vi "nanocal -- nuclear schottky fit V8.vi"() -> ()   [LabVIEW 2021] (continued)
0.000610929623   ,  \"σητS \" -> 0.000000855375   ,  \"σητN\" -> 0.000014389425    |>   , \n\"IDS0370_210908_RAW_cal__sam_\" ->   <|    \"ζ\" -> 0.013427569249   ,  \"τ1\" -> 0.019934074843   ,  \"τS\" -> 0.019524726442   ,  \"τN\" -> 0.000513623253   ,  \"τC\" -> 0.005657316251   ,  \"κ0\" -> 0.000000008143   ,  \"mm1\" -> 0.000058424467   ,  \"mm2\" -> 0.018528796956   ,  \"mm3\" -> 0.027311585694   ,  \"T\" -> 1.130000000000   ,  \"B\" -> 12.000000000000   ,  \"θ\" -> 60.000000000000   ,  \"Reoff\" -> -481927.710843376814   ,  \"Imoff\" -> 0.000000000000   ,  \"στ1\" -> 0.000000000000   ,  \"στS\" -> 0.000000000000   ,  \"στN\" -> 0.000000000000   ,  \"τ11 \" -> 0.000000000000   ,  \"τ12\" -> 0.000000000000   ,  \"τ22\" -> 0.000000000000   ,  \"τN1\" -> 0.000000000000   ,  \"τN2\" -> 0.000000000000   ,  \"σηlogτ1 \" -> 0.000000000000   ,  \"σηlogτS\" -> 0.000000000000   ,  \"σηlogτN\" -> 0.000000000000   ,  \"σlogτ1\" -> 0.000000000000   ,  \"σlogτS\" -> 0.000000000000   ,  \"σlogτN\" -> 0.000000000000   ,  \"σητ1\" -> 0.000000000000   ,  \"σητS \" -> 0.000000000000   ,  \"σητN\" -> 0.000000000000    |>   , \n\"IDS0371_210908_RAW_cal__ref_\" ->   <|    \"ζ\" -> 0.020664849580   ,  \"τ1\" -> 0.018108723176   ,  \"τS\" -> 0.010299896170   ,  \"τN\" -> 0.000079818017   ,  \"τC\" -> 0.006259144045   ,  \"κ0\" -> 0.000000013130   ,  \"mm1\" -> 0.000079811267   ,  \"mm2\" -> 0.016056535433   ,  \"mm3\" -> 0.018825729941   ,  \"T\" -> 1.900000000000   ,  \"B\" -> 12.000000000000   ,  \"θ\" -> 60.000000000000   ,  \"Reoff\" -> 0.000000000000   ,  \"Imoff\" -> 0.000000000000   ,  \"στ1\" -> 0.000000000000   ,  \"στS\" -> 0.000000000000   ,  \"στN\" -> 0.000000000000   ,  \"τ11 \" -> 0.000000000000   ,  \"τ12\" -> 0.000000000000   ,  \"τ22\" -> 0.000000000000   ,  \"τN1\" -> 0.000000000000   ,  \"τN2\" -> 0.000000000000   ,  \"σηlogτ1 \" -> 0.000000000000   ,  \"σηlogτS\" -> 0.000000000000   ,  \"σηlogτN\" -> 0.000000000000   ,  \"σlogτ1\" -> 0.000000000000   ,  \"σlogτS\" -> 0.000000000000   ,  \"σlogτN\" -> 0.000000000000   ,  \"σητ1\" -> 0.000000000000   ,  \"σητS \" -> 0.000000000000   ,  \"σητN\" -> 0.000000000000    |>   , \n\"IDS0371_210908_RAW_cal__sam_\" ->   <|    \"ζ\" -> 0.009645933094   ,  \"τ1\" -> 0.020976887035   ,  \"τS\" -> 0.013140254521   ,  \"τN\" -> 0.000215522697   ,  \"τC\" -> 0.007317042194   ,  \"κ0\" -> 0.000000013897   ,  \"mm1\" -> 0.000045154509   ,  \"mm2\" -> 0.018728618799   ,  \"mm3\" -> 0.023004762073   ,  \"T\" -> 1.900000000000   ,  \"B\" -> 12.000000000000   ,  \"θ\" -> 60.000000000000   ,  \"Reoff\" -> -120481.927710846066   ,  \"Imoff\" -> 0.000000000000   ,  \"στ1\" -> 0.000000000000   ,  \"στS\" -> 0.000000000000   ,  \"στN\" -> 0.000000000000   ,  \"τ11 \" -> 0.000000000000   ,  \"τ12\" -> 0.000000000000   ,  \"τ22\" -> 0.000000000000   ,  \"τN1\" -> 0.000000000000   ,  \"τN2\" -> 0.000000000000   ,  \"σηlogτ1 \" -> 0.000000000000   ,  \"σηlogτS\" -> 0.000000000000   ,  \"σηlogτN\" -> 0.000000000000   ,  \"σlogτ1\" -> 0.000000000000   ,  \"σlogτS\" -> 0.000000000000   ,  \"σlogτN\" -> 0.000000000000   ,  \"σητ1\" -> 0.000000000000   ,  \"σητS \" -> 0.000000000000   ,  \"σητN\" -> 0.000000000000    |>   , \n\"IDS0372_210908_RAW_cal__ref_\" ->   <|    \"ζ\" -> 0.021592146431   ,  \"τ1\" -> 0.018093446545   ,  \"τS\" -> 0.007071841556   ,  \"τN\" -> 0.000029085223   ,  \"τC\" -> 0.005341206531   ,  \"κ0\" -> 0.000000023517   ,  \"mm1\" -> 0.000065243548   ,  \"mm2\" -> 0.012435446609   ,  \"mm3\" -> 0.018188213949   ,  \"T\" -> 3.110000000000   ,  \"B\" -> 12.000000000000   ,  \"θ\" -> 60.000000000000   ,  \"Reoff\" -> 0.000000000000   ,  \"Imoff\" -> 0.000000000000   ,  \"στ1\" -> 0.000000000000   ,  \"στS\" -> 0.000000000000   ,  \"στN\" -> 0.000000000000   ,  \"τ11 \" -> 0.000000000000   ,  \"τ12\" -> 0.000000000000   ,  \"τ22\" -> 0.000000000000   ,  \"τN1\" -> 0.000000000000   ,  \"τN2\" -> 0.000000000000   ,  \"σηlogτ1 \" -> 0.000000000000   ,  \"σηlogτS\" -> 0.000000000000   ,  \"σηlogτN\" -> 0.000000000000   ,  \"σlogτ1\" -> 0.000000000000   ,  \"σlogτS\" -> 0.000000000000   ,  \"σlogτN\" -> 0.000000000000   ,  \"σητ1\" -> 0.000000000000   ,  \"σητS \" -> 0.000000000000   ,  \"σητN\" -> 0.000000000000    |>   , \n\"IDS0372_210908_RAW_cal__sam_\" ->   <|    \"ζ\" -> 0.010006554735   ,  \"τ1\" -> 0.021193289022   ,  \"τS\" -> 0.010059776467   ,  \"τN\" -> 0.000092737128   ,  \"τC\" -> 0.005619947239   ,  \"κ0\" -> 0.000000024358   ,  \"mm1\" -> 0.000035931477   ,  \"mm2\" -> 0.015490366222   ,  \"mm3\" -> 0.021541043840   ,  \"T\" -> 3.110000000000   ,  \"B\" -> 12.000000000000   ,  \"θ\" -> 60.000000000000   ,  \"Reoff\" -> -120481.927710846066   ,  \"Imoff\" -> 0.000000000000   ,  \"στ1\" -> 0.000000000000   ,  \"στS\" -> 0.000000000000   ,  \"στN\" -> 0.000000000000   ,  \"τ11 \" -> 0.000000000000   ,  \"τ12\" -> 0.000000000000   ,  \"τ22\" -> 0.000000000000   ,  \"τN1\" -> 0.000000000000   ,  \"τN2\" -> 0.000000000000   ,  \"σηlogτ1 \" -> 0.000000000000   ,  \"σηlogτS\" -> 0.000000000000   ,  \"σηlogτN\" -> 0.000000000000   ,  \"σlogτ1\" -> 0.000000000000   ,  \"σlogτS\" -> 0.000000000000   ,  \"σlogτN\" -> 0.000000000000   ,  \"σητ1\" -> 0.000000000000   ,  \"σητS \" -> 0.000000000000   ,  \"σητN\" -> 0.000000000000    |>   , \n\"IDS0373_210908_RAW_cal__ref_\" ->   <|    \"ζ\" -> 0.028148688120   ,  \"τ1\" -> 0.012706961955   ,  \"τS\" -> 0.003881518121   ,  \"τN\" -> 0.000007160132   ,  \"τC\" -> 0.004346615253   ,  \"κ0\" -> 0.000000058313   ,  \"mm1\" -> 0.000057355729   ,  \"mm2\" -> 0.008266435527   ,  \"mm3\" -> 0.012727925396   ,  \"T\" -> 5.750000000000   ,  \"B\" -> 12.000000000000   ,  \"θ\" -> 60.000000000000   ,  \"Reoff\" -> 0.000000000000   ,  \"Imoff\" -> 0.000000000000   ,  \"στ1\" -> 0.000000000000   ,  \"στS\" -> 0.000000000000   ,  \"στN\" -> 0.000000000000   ,  \"τ11 \" -> 0.000000000000   ,  \"τ12\" -> 0.000000000000   ,  \"τ22\" -> 0.000000000000   ,  \"τN1\" -> 0.000000000000   ,  \"τN2\" -> 0.000000000000   ,  \"σηlogτ1 \" -> 0.000000000000   ,  \"σηlogτS\" -> 0.000000000000   ,  \"σηlogτN\" -> 0.000000000000   ,  \"σlogτ1\" -> 0.000000000000   ,  \"σlogτS\" -> 0.000000000000   ,  \"σlogτN\" -> 0.000000000000   ,  \"σητ1\" -> 0.000000000000   ,  \"σητS \" -> 0.000000000000   ,  \"σητN\" -> 0.000000000000    |>   , \n\"IDS0373_210908_RAW_cal__sam_\" ->   <|    \"ζ\" -> 0.009383547393   ,  \"τ1\" -> 0.021616814113   ,  \"τS\" -> 0.006389723126   ,  \"τN\" -> 0.000031102862   ,  \"τC\" -> 0.004593168461   ,  \"κ0\" -> 0.000000059183   ,  \"mm1\" -> 0.000024995592   ,  \"mm2\" -> 0.010985466166   ,  \"mm3\" -> 0.021680596929   ,  \"T\" -> 5.750000000000   ,  \"B\" -> 12.000000000000   ,  \"θ\" -> 60.000000000000   ,  \"Reoff\" -> -40000.000000000000   ,  \"Imoff\" -> 0.000000000000   ,  \"στ1\" -> 0.000000000000   ,  \"στS\" -> 0.000000000000   ,  \"στN\" -> 0.000000000000   ,  \"τ11 \" -> 0.000000000000   ,  \"τ12\" -> 0.000000000000   ,  \"τ22\" -> 0.000000000000   ,  \"τN1\" -> 0.000000000000   ,  \"τN2\" -> 0.000000000000   ,  \"σηlogτ1 \" -> 0.000000000000   ,  \"σηlogτS\" -> 0.000000000000   ,  \"σηlogτN\" -> 0.000000000000   ,  \"σlogτ1\" -> 0.000000000000   ,  \"σlogτS\" -> 0.000000000000   ,  \"σlogτN\" -> 0.000000000000   ,  \"σητ1\" -> 0.000000000000   ,  \"σητS \" -> 0.000000000000   ,  \"σητN\" -> 0.000000000000    |>   , \n\"IDS0377_210909_RAW_cal__ref_\" ->   <|    \"ζ\" -> 0.246550605323   ,  \"τ1\" -> 0.063098036224   ,  \"τS\" -> 0.035636106163   ,  \"τN\" -> 0.021974547329   ,  \"τC\" -> 0.000821092988   ,  \"κ0\" -> 0.000000001041   ,  \"mm1\" -> 0.000160015882   ,  \"mm2\" -> 0.025949965723   ,  \"mm3\" -> 0.109623742590   ,  \"T\" -> 0.197000000000   ,  \"B\" -> 8.000000000000   ,  \"θ\" -> 0.000000000000   ,  \"Reoff\" -> -36382320.441988945000   ,  \"Imoff\" -> 0.000000000000   ,  \"στ1\" -> 0.000062922538   ,  \"στS\" -> 0.000014967815   ,  \"στN\" -> 0.000031670740   ,  \"τ11 \" -> 0.000000000000   ,  \"τ12\" -> 0.000000000000   ,  \"τ22\" -> 0.000000000000   ,  \"τN1\" -> 0.000000000000   ,  \"τN2\" -> 0.000000000000   ,  \"σηlogτ1 \" -> 0.000000000000   ,  \"σηlogτS\" -> 0.000000000000   ,  \"σηlogτN\" -> 0.000000000000   ,  \"σlogτ1\" -> 0.000000000000   ,  \"σlogτS\" -> 0.000000000000   ,  \"σlogτN\" -> 0.000000000000   ,  \"σητ1\" -> 0.000000000000   ,  \"σητS \" -> 0.000000000000   ,  \"σητN\" -> 0.000000000000    |>   , \n\"IDS0377_210909_RAW_cal__sam_\" ->   <|    \"ζ\" -> 0.135798490691   ,  \"τ1\" -> 0.079257563336   ,  \"τS\" -> 0.046440970443   ,  \"τN\" -> 0.031537801980   ,  \"τC\" -> 0.001434159670   ,  \"κ0\" -> 0.000000001166   ,  \"mm1\" -> 0.000167444282   ,  \"mm2\" -> 0.031002991367   ,  \"mm3\" -> 0.138089459380   ,  \"T\" -> 0.197000000000   ,  \"B\" -> 8.000000000000   ,  \"θ\" -> 0.000000000000   ,  \"Reoff\" -> -18665662.650602411500   ,  \"Imoff\" -> 0.000000000000   ,  \"στ1\" -> 0.000000000000   ,  \"στS\" -> 0.000000000000   ,  \"στN\" -> 0.000000000000   ,  \"τ11 \" -> 0.000000000000   ,  \"τ12\" -> 0.000000000000   ,  \"τ22\" -> 0.000000000000   ,  \"τN1\" -> 0.000000000000   ,  \"τN2\" -> 0.000000000000   ,  \"σηlogτ1 \" -> 0.000000000000   ,  \"σηlogτS\" -> 0.000000000000   ,  \"σηlogτN\" -> 0.000000000000   ,  \"σlogτ1\" -> 0.000000000000   ,  \"σlogτS\" -> 0.000000000000   ,  \"σlogτN\" -> 0.000000000000   ,  \"σητ1\" -> 0.000000000000   ,  \"σητS \" -> 0.000000000000   ,  \"σητN\" -> 0.000000000000    |>   , \n\"IDS0378_210909_RAW_cal__ref_\" ->   <|    \"ζ\" -> 0.463349829387   ,  \"τ1\" -> 0.074237051581   ,  \"τS\" -> 0.056120726288   ,  \"τN\" -> 0.098410853279   ,  \"τC\" -> 0.000795788528   ,  \"κ0\" -> 0.000000000406   ,  \"mm1\" -> 0.000250303134   ,  \"mm2\" -> 0.022004830152   ,  \"mm3\" -> 0.278911467417   ,  \"T\" -> 0.122000000000   ,  \"B\" -> 8.000000000000   ,  \"θ\" -> 0.000000000000   ,  \"Reoff\" -> -133680722.891566262000   ,  \"Imoff\" -> 0.000000000000   ,  \"στ1\" -> 0.000032928627   ,  \"στS\" -> 0.000022172362   ,  \"στN\" -> 0.000014961504   ,  \"τ11 \" -> 0.000000000000   ,  \"τ12\" -> 0.000000000000   ,  \"τ22\" -> 0.000000000000   ,  \"τN1\" -> 0.000000000000   ,  \"τN2\" -> 0.000000000000   ,  \"σηlogτ1 \" -> 0.000000000000   ,  \"σηlogτS\" -> 0.000000000000   ,  \"σηlogτN\" -> 0.000000000000   ,  \"σlogτ1\" -> 0.000000000000   ,  \"σlogτS\" -> 0.000000000000   ,  \"σlogτN\" -> 0.000000000000   ,  \"σητ1\" -> 0.000000000000   ,  \"σητS \" -> 0.000000000000   ,  \"σητN\" -> 0.000000000000    |>   , \n\"IDS0378_210909_RAW_cal__sam_\" ->   <|    \"ζ\" -> 0.261650469875   ,  \"τ1\" -> 0.181870145043   ,  \"τS\" -> 0.168113301561   ,  \"τN\" -> 0.186965229666   ,  \"τC\" -> 0.001543998203   ,  \"κ0\" -> 0.000000000530   ,  \"mm1\" -> 0.000318362571   ,  \"mm2\" -> 0.069029342513   ,  \"mm3\" -> 0.562051433928   ,  \"T\" -> 0.122000000000   ,  \"B\" -> 8.000000000000   ,  \"θ\" -> 0.000000000000   ,  \"Reoff\" -> -63674698.795180723100   ,  \"Imoff\" -> 0.000000000000   ,  \"στ1\" -> 0.000000000000   ,  \"στS\" -> 0.000000000000   ,  \"στN\" -> 0.000000000000   ,  \"τ11 \" -> 0.000000000000   ,  \"τ12\" -> 0.000000000000   ,  \"τ22\" -> 0.000000000000   ,  \"τN1\" -> 0.000000000000   ,  \"τN2\" -> 0.000000000000   ,  \"σηlogτ1 \" -> 0.000000000000   ,  \"σηlogτS\" -> 0.000000000000   ,  \"σηlogτN\" -> 0.000000000000   ,  \"σlogτ1\" -> 0.000000000000   ,  \"σlogτS\" -> 0.000000000000   ,  \"σlogτN\" -> 0.000000000000   ,  \"σητ1\" -> 0.000000000000   ,  \"σητS \" -> 0.000000000000   ,  \"σητN\" -> 0.000000000000    |>   , \n\"IDS0379_210909_RAW_cal__ref_\" ->   <|    \"ζ\" -> 0.425625100321   ,  \"τ1\" -> 0.068543660714   ,  \"τS\" -> 0.058744737584   ,  \"τN\" -> 0.070392227244   ,  \"τC\" -> 0.000760428296   ,  \"κ0\" -> 0.000000000614   ,  \"mm1\" -> 0.000225582014   ,  \"mm2\" -> 0.025358510497   ,  \"mm3\" -> 0.227820894937   ,  \"T\" -> 0.148000000000   ,  \"B\" -> 8.000000000000   ,  \"θ\" -> 0.000000000000   ,  \"Reoff\" -> -114874585.635359108000   ,  \"Imoff\" -> 0.000000000000   ,  \"στ1\" -> 0.000034854333   ,  \"στS\" -> 0.000021687796   ,  \"στN\" -> 0.000018077177   ,  \"τ11 \" -> 0.000000000000   ,  \"τ12\" -> 0.000000000000   ,  \"τ22\" -> 0.000000000000   ,  \"τN1\" -> 0.000000000000   ,  \"τN2\" -> 0.000000000000   ,  \"σηlogτ1 \" -> 0.000000000000   ,  \"σηlogτS\" -> 0.000000000000   ,  \"σηlogτN\" -> 0.000000000000   ,  \"σlogτ1\" -> 0.000000000000   ,  \"σlogτS\" -> 0.000000000000   ,  \"σlogτN\" -> 0.000000000000   ,  \"σητ1\" -> 0.000000000000   ,  \"σητS \" -> 0.000000000000   ,  \"σητN\" -> 0.000000000000    |>   , \n\"IDS0379_210909_RAW_cal__sam_\" ->   <|    \"ζ\" -> 0.225699737863   ,  \"τ1\" -> 0.105340283181   ,  \"τS\" -> 0.080581728797   ,  \"τN\" -> 0.103261234048   ,  \"τC\" -> 0.001367459466   ,  \"κ0\" -> 0.000000000745   ,  \"mm1\" -> 0.000248975261   ,  \"mm2\" -> 0.035515573270   ,  \"mm3\" -> 0.296279465482   ,  \"T\" -> 0.148000000000   ,  \"B\" -> 8.000000000000   ,  \"θ\" -> 0.000000000000   ,  \"Reoff\" -> -47870481.927710846100   ,  \"Imoff\" -> 0.000000000000   ,  \"στ1\" -> 0.000000000000   ,  \"στS\" -> 0.000000000000   ,  \"στN\" -> 0.000000000000   ,  \"τ11 \" -> 0.000000000000   ,  \"τ12\" -> 0.000000000000   ,  \"τ22\" -> 0.000000000000   ,  \"τN1\" -> 0.000000000000   ,  \"τN2\" -> 0.000000000000   ,  \"σηlogτ1 \" -> 0.000000000000   ,  \"σηlogτS\" -> 0.000000000000   ,  \"σηlogτN\" -> 0.000000000000   ,  \"σlogτ1\" -> 0.000000000000   ,  \"σlogτS\" -> 0.000000000000   ,  \"σlogτN\" -> 0.000000000000   ,  \"σητ1\" -> 0.000000000000   ,  \"σητS \" -> 0.000000000000   ,  \"σητN\" -> 0.000000000000    |>   , \n\"IDS0380_210909_RAW_cal__ref_\" ->   <|    \"ζ\" -> 0.296352280059   ,  \"τ1\" -> 0.061572423860   ,  \"τS\" -> 0.035048599519   ,  \"τN\" -> 0.042254612748   ,  \"τC\" -> 0.000902434218   ,  \"κ0\" -> 0.000000000747   ,  \"mm1\" -> 0.000203161456   ,  \"mm2\" -> 0.019927495587   ,  \"mm3\" -> 0.142556396514   ,  \"T\" -> 0.168000000000   ,  \"B\" -> 8.000000000000   ,  \"θ\" -> 0.000000000000   ,  \"Reoff\" -> -60285714.285714268700   ,  \"Imoff\" -> 0.000000000000   ,  \"στ1\" -> 0.000032565063   ,  \"στS\" -> 0.000015719503   ,  \"στN\" -> 0.000016419375   ,  \"τ11 \" -> 0.000000000000   ,  \"τ12\" -> 0.000000000000   ,  \"τ22\" -> 0.000000000000   ,  \"τN1\" -> 0.000000000000   ,  \"τN2\" -> 0.000000000000   ,  \"σηlogτ1 \" -> 0.000000000000   ,  \"σηlogτS\" -> 0.000000000000   ,  \"σηlogτN\" -> 0.000000000000   ,  \"σlogτ1\" -> 0.000000000000   ,  \"σlogτS\" -> 0.000000000000   ,  \"σlogτN\" -> 0.000000000000   ,  \"σητ1\" -> 0.000000000000   ,  \"σητS \" -> 0.000000000000   ,  \"σητN\" -> 0.000000000000    |>   , \n\"IDS0380_210909_RAW_cal__sam_\" ->   <|    \"ζ\" -> 0.175751625392   ,  \"τ1\" -> 0.093635045165   ,  \"τS\" -> 0.061160146348   ,  \"τN\" -> 0.068664853746   ,  \"τC\" -> 0.001317909381   ,  \"κ0\" -> 0.000000000855   ,  \"mm1\" -> 0.000193962663   ,  \"mm2\" -> 0.031705338902   ,  \"mm3\" -> 0.215695607858   ,  \"T\" -> 0.168000000000   ,  \"B\" -> 8.000000000000   ,  \"θ\" -> 0.000000000000   ,  \"Reoff\" -> -37527108.433734938500   ,  \"Imoff\" -> 0.000000000000   ,  \"στ1\" -> 0.000000000000   ,  \"στS\" -> 0.000000000000   ,  \"στN\" -> 0.000000000000   ,  \"τ11 \" -> 0.000000000000   ,  \"τ12\" -> 0.000000000000   ,  \"τ22\" -> 0.000000000000   ,  \"τN1\" -> 0.000000000000   ,  \"τN2\" -> 0.000000000000   ,  \"σηlogτ1 \" -> 0.000000000000   ,  \"σηlogτS\" -> 0.000000000000   ,  \"σηlogτN\" -> 0.000000000000   ,  \"σlogτ1\" -> 0.000000000000   ,  \"σlogτS\" -> 0.000000000000   ,  \"σlogτN\" -> 0.000000000000   ,  \"σητ1\" -> 0.000000000000   ,  \"σητS \" -> 0.000000000000   ,  \"σητN\" -> 0.000000000000    |>   , \n\"IDS0381_210909_RAW_cal__ref_\" ->   <|    \"ζ\" -> 0.135442001180   ,  \"τ1\" -> 0.054536829593   ,  \"τS\" -> 0.027242617167   ,  \"τN\" -> 0.009575045282   ,  \"τC\" -> 0.001074749120   ,  \"κ0\" -> 0.000000001354   ,  \"mm1\" -> 0.000124377738   ,  \"mm2\" -> 0.023594165009   ,  \"mm3\" -> 0.073697356296   ,  \"T\" -> 0.250000000000   ,  \"B\" -> 8.000000000000   ,  \"θ\" -> 0.000000000000   ,  \"Reoff\" -> -15819277.108433738400   ,  \"Imoff\" -> 0.000000000000   ,  \"στ1\" -> 0.000111598282   ,  \"στS\" -> 0.000013161229   ,  \"στN\" -> 0.000059063513   ,  \"τ11 \" -> 0.000000000000   ,  \"τ12\" -> 0.000000000000   ,  \"τ22\" -> 0.000000000000   ,  \"τN1\" -> 0.000000000000   ,  \"τN2\" -> 0.000000000000   ,  \"σηlogτ1 \" -> 0.000000000000   ,  \"σηlogτS\" -> 0.000000000000   ,  \"σηlogτN\" -> 0.000000000000   ,  \"σlogτ1\" -> 0.000000000000   ,  \"σlogτS\" -> 0.000000000000   ,  \"σlogτN\" -> 0.000000000000   ,  \"σητ1\" -> 0.000000000000   ,  \"σητS \" -> 0.000000000000   ,  \"σητN\" -> 0.000000000000    |>   , \n\"IDS0381_210909_RAW_cal__sam_\" ->   <|    \"ζ\" -> 0.077362618852   ,  \"τ1\" -> 0.058638638627   ,  \"τS\" -> 0.035602410157   ,  \"τN\" -> 0.012932252536   ,  \"τC\" -> 0.001722606032   ,  \"κ0\" -> 0.000000001497   ,  \"mm1\" -> 0.000118727642   ,  \"mm2\" -> 0.027585733079   ,  \"mm3\" -> 0.084946215242   ,  \"T\" -> 0.250000000000   ,  \"B\" -> 8.000000000000   ,  \"θ\" -> 0.000000000000   ,  \"Reoff\" -> -9843373.493975907570   ,  \"Imoff\" -> 0.000000000000   ,  \"στ1\" -> 0.000000000000   ,  \"στS\" -> 0.000000000000   ,  \"στN\" -> 0.000000000000   ,  \"τ11 \" -> 0.000000000000   ,  \"τ12\" -> 0.000000000000   ,  \"τ22\" -> 0.000000000000   ,  \"τN1\" -> 0.000000000000   ,  \"τN2\" -> 0.000000000000   ,  \"σηlogτ1 \" -> 0.000000000000   ,  \"σηlogτS\" -> 0.000000000000   ,  \"σηlogτN\" -> 0.000000000000   ,  \"σlogτ1\" -> 0.000000000000   ,  \"σlogτS\" -> 0.000000000000   ,  \"σlogτN\" -> 0.000000000000   ,  \"σητ1\" -> 0.000000000000   ,  \"σητS \" -> 0.000000000000   ,  \"σητN\" -> 0.000000000000    |>   , \n\"IDS0382_210909_RAW_cal__ref_\" ->   <|    \"ζ\" -> 0.083327700805   ,  \"τ1\" -> 0.049870021008   ,  \"τS\" -> 0.024726462582   ,  \"τN\" -> 0.005137571358   ,  \"τC\" -> 0.001213133652   ,  \"κ0\" -> 0.000000001736   ,  \"mm1\" -> 0.000089554374   ,  \"mm2\" -> 0.023106179536   ,  \"mm3\" -> 0.060239955976   ,  \"T\" -> 0.300000000000   ,  \"B\" -> 8.000000000000   ,  \"θ\" -> 0.000000000000   ,  \"Reoff\" -> -7659638.554216861730   ,  \"Imoff\" -> 0.000000000000   ,  \"στ1\" -> 0.000221537334   ,  \"στS\" -> 0.000014924990   ,  \"στN\" -> 0.000118586370   ,  \"τ11 \" -> 0.000000000000   ,  \"τ12\" -> 0.000000000000   ,  \"τ22\" -> 0.000000000000   ,  \"τN1\" -> 0.000000000000   ,  \"τN2\" -> 0.000000000000   ,  \"σηlogτ1 \" -> 0.000000000000   ,  \"σηlogτS\" -> 0.000000000000   ,  \"σηlogτN\" -> 0.000000000000   ,  \"σlogτ1\" -> 0.000000000000   ,  \"σlogτS\" -> 0.000000000000   ,  \"σlogτN\" -> 0.000000000000   ,  \"σητ1\" -> 0.000000000000   ,  \"σητS \" -> 0.000000000000   ,  \"σητN\" -> 0.000000000000    |>   , \n\"IDS0382_210909_RAW_cal__sam_\" ->   <|    \"ζ\" -> 0.054029770351   ,  \"τ1\" -> 0.051440847518   ,  \"τS\" -> 0.032079834642   ,  \"τN\" -> 0.007150632998   ,  \"τC\" -> 0.002202148776   ,  \"κ0\" -> 0.000000001884   ,  \"mm1\" -> 0.000106291219   ,  \"mm2\" -> 0.027352636275   ,  \"mm3\" -> 0.067534149597   ,  \"T\" -> 0.300000000000   ,  \"B\" -> 8.000000000000   ,  \"θ\" -> 0.000000000000   ,  \"Reoff\" -> 0.000000000000   ,  \"Imoff\" -> 0.000000000000   ,  \"στ1\" -> 0.000000000000   ,  \"στS\" -> 0.000000000000   ,  \"στN\" -> 0.000000000000   ,  \"τ11 \" -> 0.000000000000   ,  \"τ12\" -> 0.000000000000   ,  \"τ22\" -> 0.000000000000   ,  \"τN1\" -> 0.000000000000   ,  \"τN2\" -> 0.000000000000   ,  \"σηlogτ1 \" -> 0.000000000000   ,  \"σηlogτS\" -> 0.000000000000   ,  \"σηlogτN\" -> 0.000000000000   ,  \"σlogτ1\" -> 0.000000000000   ,  \"σlogτS\" -> 0.000000000000   ,  \"σlogτN\" -> 0.000000000000   ,  \"σητ1\" -> 0.000000000000   ,  \"σητS \" -> 0.000000000000   ,  \"σητN\" -> 0.000000000000    |>   , \n\"IDS0383_210910_RAW_cal__ref_\" ->   <|    \"ζ\" -> 0.062724752087   ,  \"τ1\" -> 0.048607141774   ,  \"τS\" -> 0.023827543799   ,  \"τN\" -> 0.003390848411   ,  \"τC\" -> 0.001761568500   ,  \"κ0\" -> 0.000000002107   ,  \"mm1\" -> 0.000097559485   ,  \"mm2\" -> 0.023589285914   ,  \"mm3\" -> 0.055607523989   ,  \"T\" -> 0.360000000000   ,  \"B\" -> 8.000000000000   ,  \"θ\" -> 0.000000000000   ,  \"Reoff\" -> -3448979.591836734680   ,  \"Imoff\" -> 0.000000000000   ,  \"στ1\" -> 0.000376669141   ,  \"στS\" -> 0.000017301947   ,  \"στN\" -> 0.000201176295   ,  \"τ11 \" -> 0.000000000000   ,  \"τ12\" -> 0.000000000000   ,  \"τ22\" -> 0.000000000000   ,  \"τN1\" -> 0.000000000000   ,  \"τN2\" -> 0.000000000000   ,  \"σηlogτ1 \" -> 0.000000000000   ,  \"σηlogτS\" -> 0.000000000000   ,  \"σηlogτN\" -> 0.000000000000   ,  \"σlogτ1\" -> 0.000000000000   ,  \"σlogτS\" -> 0.000000000000   ,  \"σlogτN\" -> 0.000000000000   ,  \"σητ1\" -> 0.000000000000   ,  \"σητS \" -> 0.000000000000   ,  \"σητN\" -> 0.000000000000    |>   , \n\"IDS0383_210910_RAW_cal__sam_\" ->   <|    \"ζ\" -> 0.038341835326   ,  \"τ1\" -> 0.050866858713   ,  \"τS\" -> 0.030652081909   ,  \"τN\" -> 0.004623805952   ,  \"τC\" -> 0.002823684758   ,  \"κ0\" -> 0.000000002289   ,  \"mm1\" -> 0.000096034779   ,  \"mm2\" -> 0.028459102290   ,  \"mm3\" -> 0.061763836547   ,  \"T\" -> 0.360000000000   ,  \"B\" -> 8.000000000000   ,  \"θ\" -> 0.000000000000   ,  \"Reoff\" -> 0.000000000000   ,  \"Imoff\" -> 0.000000000000   ,  \"στ1\" -> 0.000000000000   ,  \"στS\" -> 0.000000000000   ,  \"στN\" -> 0.000000000000   ,  \"τ11 \" -> 0.000000000000   ,  \"τ12\" -> 0.000000000000   ,  \"τ22\" -> 0.000000000000   ,  \"τN1\" -> 0.000000000000   ,  \"τN2\" -> 0.000000000000   ,  \"σηlogτ1 \" -> 0.000000000000   ,  \"σηlogτS\" -> 0.000000000000   ,  \"σηlogτN\" -> 0.000000000000   ,  \"σlogτ1\" -> 0.000000000000   ,  \"σlogτS\" -> 0.000000000000   ,  \"σlogτN\" -> 0.000000000000   ,  \"σητ1\" -> 0.000000000000   ,  \"σητS \" -> 0.000000000000   ,  \"σητN\" -> 0.000000000000    |>   , \n\"IDS0384_210910_RAW_cal__ref_\" ->   <|    \"ζ\" -> 0.048414028377   ,  \"τ1\" -> 0.045010611313   ,  \"τS\" -> 0.024057574241   ,  \"τN\" -> 0.002275401127   ,  \"τC\" -> 0.001753445489   ,  \"κ0\" -> 0.000000002628   ,  \"mm1\" -> 0.000075920940   ,  \"mm2\" -> 0.024140914114   ,  \"mm3\" -> 0.050155082533   ,  \"T\" -> 0.430000000000   ,  \"B\" -> 8.000000000000   ,  \"θ\" -> 0.000000000000   ,  \"Reoff\" -> -3244897.959183673380   ,  \"Imoff\" -> 0.000000000000   ,  \"στ1\" -> 0.000665063032   ,  \"στS\" -> 0.000021368158   ,  \"στN\" -> 0.000342578343   ,  \"τ11 \" -> 0.000000000000   ,  \"τ12\" -> 0.000000000000   ,  \"τ22\" -> 0.000000000000   ,  \"τN1\" -> 0.000000000000   ,  \"τN2\" -> 0.000000000000   ,  \"σηlogτ1 \" -> 0.000000000000   ,  \"σηlogτS\" -> 0.000000000000   ,  \"σηlogτN\" -> 0.000000000000   ,  \"σlogτ1\" -> 0.000000000000   ,  \"σlogτS\" -> 0.000000000000   ,  \"σlogτN\" -> 0.000000000000   ,  \"σητ1\" -> 0.000000000000   ,  \"σητS \" -> 0.000000000000   ,  \"σητN\" -> 0.000000000000    |>   , \n\"IDS0384_210910_RAW_cal__sam_\" ->   <|    \"ζ\" -> 0.029950572027   ,  \"τ1\" -> 0.044923259835   ,  \"τS\" -> 0.030416367718   ,  \"τN\" -> 0.002541256331   ,  \"τC\" -> 0.003331031560   ,  \"κ0\" -> 0.000000002858   ,  \"mm1\" -> 0.000087776347   ,  \"mm2\" -> 0.029544080465   ,  \"mm3\" -> 0.052567158325   ,  \"T\" -> 0.430000000000   ,  \"B\" -> 8.000000000000   ,  \"θ\" -> 0.000000000000   ,  \"Reoff\" -> 0.000000000000   ,  \"Imoff\" -> 0.000000000000   ,  \"στ1\" -> 0.000000000000   ,  \"στS\" -> 0.000000000000   ,  \"στN\" -> 0.000000000000   ,  \"τ11 \" -> 0.000000000000   ,  \"τ12\" -> 0.000000000000   ,  \"τ22\" -> 0.000000000000   ,  \"τN1\" -> 0.000000000000   ,  \"τN2\" -> 0.000000000000   ,  \"σηlogτ1 \" -> 0.000000000000   ,  \"σηlogτS\" -> 0.000000000000   ,  \"σηlogτN\" -> 0.000000000000   ,  \"σlogτ1\" -> 0.000000000000   ,  \"σlogτS\" -> 0.000000000000   ,  \"σlogτN\" -> 0.000000000000   ,  \"σητ1\" -> 0.000000000000   ,  \"σητS \" -> 0.000000000000   ,  \"σητN\" -> 0.000000000000    |>   , \n\"IDS0385_210910_RAW_cal__ref_\" ->   <|    \"ζ\" -> 0.037803233744   ,  \"τ1\" -> 0.038048590559   ,  \"τS\" -> 0.025073667725   ,  \"τN\" -> 0.001214857209   ,  \"τC\" -> 0.002021423784   ,  \"κ0\" -> 0.000000003274   ,  \"mm1\" -> 0.000068491984   ,  \"mm2\" -> 0.025433188254   ,  \"mm3\" -> 0.041850650292   ,  \"T\" -> 0.530000000000   ,  \"B\" -> 8.000000000000   ,  \"θ\" -> 0.000000000000   ,  \"Reoff\" -> -1979591.836734693500   ,  \"Imoff\" -> 0.000000000000   ,  \"στ1\" -> 0.001496353936   ,  \"στS\" -> 0.000028774209   ,  \"στN\" -> 0.000698641170   ,  \"τ11 \" -> 0.000000000000   ,  \"τ12\" -> 0.000000000000   ,  \"τ22\" -> 0.000000000000   ,  \"τN1\" -> 0.000000000000   ,  \"τN2\" -> 0.000000000000   ,  \"σηlogτ1 \" -> 0.000000000000   ,  \"σηlogτS\" -> 0.000000000000   ,  \"σηlogτN\" -> 0.000000000000   ,  \"σlogτ1\" -> 0.000000000000   ,  \"σlogτS\" -> 0.000000000000   ,  \"σlogτN\" -> 0.000000000000   ,  \"σητ1\" -> 0.000000000000   ,  \"σητS \" -> 0.000000000000   ,  \"σητN\" -> 0.000000000000    |>   , \n\"IDS0385_210910_RAW_cal__sam_\" ->   <|    \"ζ\" -> 0.024600756648   ,  \"τ1\" -> 0.043958236582   ,  \"τS\" -> 0.031312750224   ,  \"τN\" -> 0.001348105931   ,  \"τC\" -> 0.003635120795   ,  \"κ0\" -> 0.000000003548   ,  \"mm1\" -> 0.000078569164   ,  \"mm2\" -> 0.031960914170   ,  \"mm3\" -> 0.049018211972   ,  \"T\" -> 0.530000000000   ,  \"B\" -> 8.000000000000   ,  \"θ\" -> 0.000000000000   ,  \"Reoff\" -> 0.000000000000   ,  \"Imoff\" -> 0.000000000000   ,  \"στ1\" -> 0.000000000000   ,  \"στS\" -> 0.000000000000   ,  \"στN\" -> 0.000000000000   ,  \"τ11 \" -> 0.000000000000   ,  \"τ12\" -> 0.000000000000   ,  \"τ22\" -> 0.000000000000   ,  \"τN1\" -> 0.000000000000   ,  \"τN2\" -> 0.000000000000   ,  \"σηlogτ1 \" -> 0.000000000000   ,  \"σηlogτS\" -> 0.000000000000   ,  \"σηlogτN\" -> 0.000000000000   ,  \"σlogτ1\" -> 0.000000000000   ,  \"σlogτS\" -> 0.000000000000   ,  \"σlogτN\" -> 0.000000000000   ,  \"σητ1\" -> 0.000000000000   ,  \"σητS \" -> 0.000000000000   ,  \"σητN\" -> 0.000000000000    |>   , \n\"IDS0386_210910_RAW_cal__ref_\" ->   <|    \"ζ\" -> 0.027746649612   ,  \"τ1\" -> 0.033747008640   ,  \"τS\" -> 0.026895844648   ,  \"τN\" -> 0.000802809162   ,  \"τC\" -> 0.002381968002   ,  \"κ0\" -> 0.000000003893   ,  \"mm1\" -> 0.000059322452   ,  \"mm2\" -> 0.026788808143   ,  \"mm3\" -> 0.037748044699   ,  \"T\" -> 0.630000000000   ,  \"B\" -> 8.000000000000   ,  \"θ\" -> 0.000000000000   ,  \"Reoff\" -> -918367.346938774919   ,  \"Imoff\" -> 0.000000000000   ,  \"στ1\" -> 0.002776813512   ,  \"στS\" -> 0.000037245612   ,  \"στN\" -> 0.001225903353   ,  \"τ11 \" -> 0.000000000000   ,  \"τ12\" -> 0.000000000000   ,  \"τ22\" -> 0.000000000000   ,  \"τN1\" -> 0.000000000000   ,  \"τN2\" -> 0.000000000000   ,  \"σηlogτ1 \" -> 0.000000000000   ,  \"σηlogτS\" -> 0.000000000000   ,  \"σηlogτN\" -> 0.000000000000   ,  \"σlogτ1\" -> 0.000000000000   ,  \"σlogτS\" -> 0.000000000000   ,  \"σlogτN\" -> 0.000000000000   ,  \"σητ1\" -> 0.000000000000   ,  \"σητS \" -> 0.000000000000   ,  \"σητN\" -> 0.000000000000    |>   , \n\"IDS0386_210910_RAW_cal__sam_\" ->   <|    \"ζ\" -> 0.019494767421   ,  \"τ1\" -> 0.040349410363   ,  \"τS\" -> 0.033202805363   ,  \"τN\" -> 0.000770756985   ,  \"τC\" -> 0.004303152006   ,  \"κ0\" -> 0.000000004241   ,  \"mm1\" -> 0.000073144130   ,  \"mm2\" -> 0.033928832906   ,  \"mm3\" -> 0.045286454378   ,  \"T\" -> 0.630000000000   ,  \"B\" -> 8.000000000000   ,  \"θ\" -> 0.000000000000   ,  \"Reoff\" -> 0.000000000000   ,  \"Imoff\" -> 0.000000000000   ,  \"στ1\" -> 0.000000000000   ,  \"στS\" -> 0.000000000000   ,  \"στN\" -> 0.000000000000   ,  \"τ11 \" -> 0.000000000000   ,  \"τ12\" -> 0.000000000000   ,  \"τ22\" -> 0.000000000000   ,  \"τN1\" -> 0.000000000000   ,  \"τN2\" -> 0.000000000000   ,  \"σηlogτ1 \" -> 0.000000000000   ,  \"σηlogτS\" -> 0.000000000000   ,  \"σηlogτN\" -> 0.000000000000   ,  \"σlogτ1\" -> 0.000000000000   ,  \"σlogτS\" -> 0.000000000000   ,  \"σlogτN\" -> 0.000000000000   ,  \"σητ1\" -> 0.000000000000   ,  \"σητS \" -> 0.000000000000   ,  \"σητN\" -> 0.000000000000    |>   , \n\"IDS0387_210910_RAW_cal__ref_\" ->   <|    \"ζ\" -> 0.019313601846   ,  \"τ1\" -> 0.030127940029   ,  \"τS\" -> 0.030834079671   ,  \"τN\" -> 0.000314036282   ,  \"τC\" -> 0.003752610189   ,  \"κ0\" -> 0.000000005418   ,  \"mm1\" -> 0.000063634095   ,  \"mm2\" -> 0.028697652257   ,  \"mm3\" -> 0.036868962129   ,  \"T\" -> 0.830000000000   ,  \"B\" -> 8.000000000000   ,  \"θ\" -> 0.000000000000   ,  \"Reoff\" -> -265306.122448978945   ,  \"Imoff\" -> 0.000000000000   ,  \"στ1\" -> 0.011424377975   ,  \"στS\" -> 0.000061541841   ,  \"στN\" -> 0.005052534408   ,  \"τ11 \" -> 0.000000000000   ,  \"τ12\" -> 0.000000000000   ,  \"τ22\" -> 0.000000000000   ,  \"τN1\" -> 0.000000000000   ,  \"τN2\" -> 0.000000000000   ,  \"σηlogτ1 \" -> 0.000000000000   ,  \"σηlogτS\" -> 0.000000000000   ,  \"σηlogτN\" -> 0.000000000000   ,  \"σlogτ1\" -> 0.000000000000   ,  \"σlogτS\" -> 0.000000000000   ,  \"σlogτN\" -> 0.000000000000   ,  \"σητ1\" -> 0.000000000000   ,  \"σητS \" -> 0.000000000000   ,  \"σητN\" -> 0.000000000000    |>   , \n\"IDS0387_210910_RAW_cal__sam_\" ->   <|    \"ζ\" -> 0.013958531253   ,  \"τ1\" -> 0.040449551738   ,  \"τS\" -> 0.038075316972   ,  \"τN\" -> 0.000218997482   ,  \"τC\" -> 0.005348147372   ,  \"κ0\" -> 0.000000005866   ,  \"mm1\" -> 0.000064761782   ,  \"mm2\" -> 0.038768935960   ,  \"mm3\" -> 0.045792848207   ,  \"T\" -> 0.830000000000   ,  \"B\" -> 8.000000000000   ,  \"θ\" -> 0.000000000000   ,  \"Reoff\" -> 0.000000000000   ,  \"Imoff\" -> 0.000000000000   ,  \"στ1\" -> 0.000000000000   ,  \"στS\" -> 0.000000000000   ,  \"στN\" -> 0.000000000000   ,  \"τ11 \" -> 0.000000000000   ,  \"τ12\" -> 0.000000000000   ,  \"τ22\" -> 0.000000000000   ,  \"τN1\" -> 0.000000000000   ,  \"τN2\" -> 0.000000000000   ,  \"σηlogτ1 \" -> 0.000000000000   ,  \"σηlogτS\" -> 0.000000000000   ,  \"σηlogτN\" -> 0.000000000000   ,  \"σlogτ1\" -> 0.000000000000   ,  \"σlogτS\" -> 0.000000000000   ,  \"σlogτN\" -> 0.000000000000   ,  \"σητ1\" -> 0.000000000000   ,  \"σητS \" -> 0.000000000000   ,  \"σητN\" -> 0.000000000000    |>   , \n\"IDS0388_210910_RAW_cal__ref_\" ->   <|    \"ζ\" -> 0.016319215592   ,  \"τ1\" -> 0.028476907475   ,  \"τS\" -> 0.040634863110   ,  \"τN\" -> 0.000119778793   ,  \"τC\" -> 0.003363489331   ,  \"κ0\" -> 0.000000007540   ,  \"mm1\" -> 0.000049996694   ,  \"mm2\" -> 0.028266417043   ,  \"mm3\" -> 0.044943708759   ,  \"T\" -> 1.130000000000   ,  \"B\" -> 8.000000000000   ,  \"θ\" -> 0.000000000000   ,  \"Reoff\" -> -428571.428571428172   ,  \"Imoff\" -> 0.000000000000   ,  \"στ1\" -> 0.056097814520   ,  \"στS\" -> 0.000101338732   ,  \"στN\" -> 0.027741009439   ,  \"τ11 \" -> 0.000000000000   ,  \"τ12\" -> 0.000000000000   ,  \"τ22\" -> 0.000000000000   ,  \"τN1\" -> 0.000000000000   ,  \"τN2\" -> 0.000000000000   ,  \"σηlogτ1 \" -> 0.000000000000   ,  \"σηlogτS\" -> 0.000000000000   ,  \"σηlogτN\" -> 0.000000000000   ,  \"σlogτ1\" -> 0.000000000000   ,  \"σlogτS\" -> 0.000000000000   ,  \"σlogτN\" -> 0.000000000000   ,  \"σητ1\" -> 0.000000000000   ,  \"σητS \" -> 0.000000000000   ,  \"σητN\" -> 0.000000000000    |>   , \n\"IDS0388_210910_RAW_cal__sam_\" ->   <|    \"ζ\" -> 0.011551866824   ,  \"τ1\" -> 0.040411227639   ,  \"τS\" -> 0.048181354691   ,  \"τN\" -> 0.000103559724   ,  \"τC\" -> 0.006232382617   ,  \"κ0\" -> 0.000000008161   ,  \"mm1\" -> 0.000063176601   ,  \"mm2\" -> 0.040126882627   ,  \"mm3\" -> 0.055296246344   ,  \"T\" -> 1.130000000000   ,  \"B\" -> 8.000000000000   ,  \"θ\" -> 0.000000000000   ,  \"Reoff\" -> 0.000000000000   ,  \"Imoff\" -> 0.000000000000   ,  \"στ1\" -> 0.000000000000   ,  \"στS\" -> 0.000000000000   ,  \"στN\" -> 0.000000000000   ,  \"τ11 \" -> 0.000000000000   ,  \"τ12\" -> 0.000000000000   ,  \"τ22\" -> 0.000000000000   ,  \"τN1\" -> 0.000000000000   ,  \"τN2\" -> 0.000000000000   ,  \"σηlogτ1 \" -> 0.000000000000   ,  \"σηlogτS\" -> 0.000000000000   ,  \"σηlogτN\" -> 0.000000000000   ,  \"σlogτ1\" -> 0.000000000000   ,  \"σlogτS\" -> 0.000000000000   ,  \"σlogτN\" -> 0.000000000000   ,  \"σητ1\" -> 0.000000000000   ,  \"σητS \" -> 0.000000000000   ,  \"σητN\" -> 0.000000000000    |>   , \n\"IDS0389_210910_RAW_cal__ref_\" ->   <|    \"ζ\" -> 0.019598304636   ,  \"τ1\" -> 0.026919422871   ,  \"τS\" -> 0.016301457757   ,  \"τN\" -> 0.000045685674   ,  \"τC\" -> 0.003967911941   ,  \"κ0\" -> 0.000000010417   ,  \"mm1\" -> 0.000061755971   ,  \"mm2\" -> 0.020381971483   ,  \"mm3\" -> 0.027111127086   ,  \"T\" -> 1.520000000000   ,  \"B\" -> 8.000000000000   ,  \"θ\" -> 0.000000000000   ,  \"Reoff\" -> -551020.408163265324   ,  \"Imoff\" -> 0.000000000000   ,  \"στ1\" -> 0.092677427953   ,  \"στS\" -> 0.000105745650   ,  \"στN\" -> 0.043266676347   ,  \"τ11 \" -> 0.000000000000   ,  \"τ12\" -> 0.000000000000   ,  \"τ22\" -> 0.000000000000   ,  \"τN1\" -> 0.000000000000   ,  \"τN2\" -> 0.000000000000   ,  \"σηlogτ1 \" -> 0.000000000000   ,  \"σηlogτS\" -> 0.000000000000   ,  \"σηlogτN\" -> 0.000000000000   ,  \"σlogτ1\" -> 0.000000000000   ,  \"σlogτS\" -> 0.000000000000   ,  \"σlogτN\" -> 0.000000000000   ,  \"σητ1\" -> 0.000000000000   ,  \"σητS \" -> 0.000000000000   ,  \"σητN\" -> 0.000000000000    |>   , \n\"IDS0389_210910_RAW_cal__sam_\" ->   <|    \"ζ\" -> 0.011148198813   ,  \"τ1\" -> 0.038849151842   ,  \"τS\" -> 0.019213865355   ,  \"τN\" -> 0.000045035153   ,  \"τC\" -> 0.005536708133   ,  \"κ0\" -> 0.000000011229   ,  \"mm1\" -> 0.000047596165   ,  \"mm2\" -> 0.024836509281   ,  \"mm3\" -> 0.038975357089   ,  \"T\" -> 1.520000000000   ,  \"B\" -> 8.000000000000   ,  \"θ\" -> 0.000000000000   ,  \"Reoff\" -> 0.000000000000   ,  \"Imoff\" -> 0.000000000000   ,  \"στ1\" -> 0.000000000000   ,  \"στS\" -> 0.000000000000   ,  \"στN\" -> 0.000000000000   ,  \"τ11 \" -> 0.000000000000   ,  \"τ12\" -> 0.000000000000   ,  \"τ22\" -> 0.000000000000   ,  \"τN1\" -> 0.000000000000   ,  \"τN2\" -> 0.000000000000   ,  \"σηlogτ1 \" -> 0.000000000000   ,  \"σηlogτS\" -> 0.000000000000   ,  \"σηlogτN\" -> 0.000000000000   ,  \"σlogτ1\" -> 0.000000000000   ,  \"σlogτS\" -> 0.000000000000   ,  \"σlogτN\" -> 0.000000000000   ,  \"σητ1\" -> 0.000000000000   ,  \"σητS \" -> 0.000000000000   ,  \"σητN\" -> 0.000000000000    |>   , \n\"IDS0390_210910_RAW_cal__ref_\" ->   <|    \"ζ\" -> 0.016930911493   ,  \"τ1\" -> 0.024035041541   ,  \"τS\" -> 0.011182752166   ,  \"τN\" -> 0.000024854278   ,  \"τC\" -> 0.003445627696   ,  \"κ0\" -> 0.000000013051   ,  \"mm1\" -> 0.000044158259   ,  \"mm2\" -> 0.014733556006   ,  \"mm3\" -> 0.024100316408   ,  \"T\" -> 1.900000000000   ,  \"B\" -> 8.000000000000   ,  \"θ\" -> 0.000000000000   ,  \"Reoff\" -> -346938.775510204024   ,  \"Imoff\" -> 0.000000000000   ,  \"στ1\" -> 0.156695414704   ,  \"στS\" -> 0.000120966838   ,  \"στN\" -> 0.078791038522   ,  \"τ11 \" -> 0.000000000000   ,  \"τ12\" -> 0.000000000000   ,  \"τ22\" -> 0.000000000000   ,  \"τN1\" -> 0.000000000000   ,  \"τN2\" -> 0.000000000000   ,  \"σηlogτ1 \" -> 0.000000000000   ,  \"σηlogτS\" -> 0.000000000000   ,  \"σηlogτN\" -> 0.000000000000   ,  \"σlogτ1\" -> 0.000000000000   ,  \"σlogτS\" -> 0.000000000000   ,  \"σlogτN\" -> 0.000000000000   ,  \"σητ1\" -> 0.000000000000   ,  \"σητS \" -> 0.000000000000   ,  \"σητN\" -> 0.000000000000    |>   , \n\"IDS0390_210910_RAW_cal__sam_\" ->   <|    \"ζ\" -> 0.010826949430   ,  \"τ1\" -> 0.038768037521   ,  \"τS\" -> 0.012925317198   ,  \"τN\" -> 0.000029157336   ,  \"τC\" -> 0.005196063884   ,  \"κ0\" -> 0.000000013864   ,  \"mm1\" -> 0.000039906108   ,  \"mm2\" -> 0.018195372076   ,  \"mm3\" -> 0.038823555195   ,  \"T\" -> 1.900000000000   ,  \"B\" -> 8.000000000000   ,  \"θ\" -> 0.000000000000   ,  \"Reoff\" -> 0.000000000000   ,  \"Imoff\" -> 0.000000000000   ,  \"στ1\" -> 0.000000000000   ,  \"στS\" -> 0.000000000000   ,  \"στN\" -> 0.000000000000   ,  \"τ11 \" -> 0.000000000000   ,  \"τ12\" -> 0.000000000000   ,  \"τ22\" -> 0.000000000000   ,  \"τN1\" -> 0.000000000000   ,  \"τN2\" -> 0.000000000000   ,  \"σηlogτ1 \" -> 0.000000000000   ,  \"σηlogτS\" -> 0.000000000000   ,  \"σηlogτN\" -> 0.000000000000   ,  \"σlogτ1\" -> 0.000000000000   ,  \"σlogτS\" -> 0.000000000000   ,  \"σlogτN\" -> 0.000000000000   ,  \"σητ1\" -> 0.000000000000   ,  \"σητS \" -> 0.000000000000   ,  \"σητN\" -> 0.000000000000    |>   , \n\"IDS0391_210910_RAW_cal__ref_\" ->   <|    \"ζ\" -> 0.014199379988   ,  \"τ1\" -> 0.031876047451   ,  \"τS\" -> 0.042500159356   ,  \"τN\" -> 0.000092944151   ,  \"τC\" -> 0.003599424306   ,  \"κ0\" -> 0.000000008340   ,  \"mm1\" -> 0.000046556540   ,  \"mm2\" -> 0.031676737878   ,  \"mm3\" -> 0.046950076508   ,  \"T\" -> 1.250000000000   ,  \"B\" -> 8.000000000000   ,  \"θ\" -> 0.000000000000   ,  \"Reoff\" -> -224489.795918366871   ,  \"Imoff\" -> 0.000000000000   ,  \"στ1\" -> 0.081986423861   ,  \"στS\" -> 0.000106847397   ,  \"στN\" -> 0.039114279615   ,  \"τ11 \" -> 0.000000000000   ,  \"τ12\" -> 0.000000000000   ,  \"τ22\" -> 0.000000000000   ,  \"τN1\" -> 0.000000000000   ,  \"τN2\" -> 0.000000000000   ,  \"σηlogτ1 \" -> 0.000000000000   ,  \"σηlogτS\" -> 0.000000000000   ,  \"σηlogτN\" -> 0.000000000000   ,  \"σlogτ1\" -> 0.000000000000   ,  \"σlogτS\" -> 0.000000000000   ,  \"σlogτN\" -> 0.000000000000   ,  \"σητ1\" -> 0.000000000000   ,  \"σητS \" -> 0.000000000000   ,  \"σητN\" -> 0.000000000000    |>   , \n\"IDS0391_210910_RAW_cal__sam_\" ->   <|    \"ζ\" -> 0.010962610928   ,  \"τ1\" -> 0.040398807374   ,  \"τS\" -> 0.051328988590   ,  \"τN\" -> 0.000070281011   ,  \"τC\" -> 0.006422533164   ,  \"κ0\" -> 0.000000008958   ,  \"mm1\" -> 0.000062039854   ,  \"mm2\" -> 0.040240103995   ,  \"mm3\" -> 0.058481936484   ,  \"T\" -> 1.250000000000   ,  \"B\" -> 8.000000000000   ,  \"θ\" -> 0.000000000000   ,  \"Reoff\" -> 0.000000000000   ,  \"Imoff\" -> 0.000000000000   ,  \"στ1\" -> 0.000000000000   ,  \"στS\" -> 0.000000000000   ,  \"στN\" -> 0.000000000000   ,  \"τ11 \" -> 0.000000000000   ,  \"τ12\" -> 0.000000000000   ,  \"τ22\" -> 0.000000000000   ,  \"τN1\" -> 0.000000000000   ,  \"τN2\" -> 0.000000000000   ,  \"σηlogτ1 \" -> 0.000000000000   ,  \"σηlogτS\" -> 0.000000000000   ,  \"σηlogτN\" -> 0.000000000000   ,  \"σlogτ1\" -> 0.000000000000   ,  \"σlogτS\" -> 0.000000000000   ,  \"σlogτN\" -> 0.000000000000   ,  \"σητ1\" -> 0.000000000000   ,  \"σητS \" -> 0.000000000000   ,  \"σητN\" -> 0.000000000000    |>   , \n\"IDS0392_210910_RAW_cal__ref_\" ->   <|    \"ζ\" -> 0.015881193155   ,  \"τ1\" -> 0.030137709791   ,  \"τS\" -> 0.030744706039   ,  \"τN\" -> 0.000065162997   ,  \"τC\" -> 0.003875572630   ,  \"κ0\" -> 0.000000009446   ,  \"mm1\" -> 0.000053981464   ,  \"mm2\" -> 0.029765266989   ,  \"mm3\" -> 0.035493200486   ,  \"T\" -> 1.390000000000   ,  \"B\" -> 8.000000000000   ,  \"θ\" -> 0.000000000000   ,  \"Reoff\" -> -224489.795918366871   ,  \"Imoff\" -> 0.000000000000   ,  \"στ1\" -> 0.096426784918   ,  \"στS\" -> 0.000107023117   ,  \"στN\" -> 0.042599463915   ,  \"τ11 \" -> 0.000000000000   ,  \"τ12\" -> 0.000000000000   ,  \"τ22\" -> 0.000000000000   ,  \"τN1\" -> 0.000000000000   ,  \"τN2\" -> 0.000000000000   ,  \"σηlogτ1 \" -> 0.000000000000   ,  \"σηlogτS\" -> 0.000000000000   ,  \"σηlogτN\" -> 0.000000000000   ,  \"σlogτ1\" -> 0.000000000000   ,  \"σlogτS\" -> 0.000000000000   ,  \"σlogτN\" -> 0.000000000000   ,  \"σητ1\" -> 0.000000000000   ,  \"σητS \" -> 0.000000000000   ,  \"σητN\" -> 0.000000000000    |>   , \n\"IDS0392_210910_RAW_cal__sam_\" ->   <|    \"ζ\" -> 0.010962610928   ,  \"τ1\" -> 0.040398807374   ,  \"τS\" -> 0.051328988590   ,  \"τN\" -> 0.000070281011   ,  \"τC\" -> 0.006422533164   ,  \"κ0\" -> 0.000000008958   ,  \"mm1\" -> 0.000062039854   ,  \"mm2\" -> 0.040240103995   ,  \"mm3\" -> 0.058481936484   ,  \"T\" -> 1.390000000000   ,  \"B\" -> 8.000000000000   ,  \"θ\" -> 0.000000000000   ,  \"Reoff\" -> 0.000000000000   ,  \"Imoff\" -> 0.000000000000   ,  \"στ1\" -> 0.000000000000   ,  \"στS\" -> 0.000000000000   ,  \"στN\" -> 0.000000000000   ,  \"τ11 \" -> 0.000000000000   ,  
